vi "Create Actor Object.vi"(8 "error in (no error)":errorcluster, 10 "Object Name":string, 11 "CS++Factory in":refnum<class "CS++Factory.lvclass">) -> (0 "error out":errorcluster, 1 "Attributes found?":bool, 2 "C++BaseActor":refnum<class "CS++BaseActor.lvclass">, 3 "CS++Factory out":refnum<class "CS++Factory.lvclass">)   [LabVIEW 2013, in "CS++BaseClasses.lvlib" / "CS++Factory.lvclass"]
doc: "Create an actor object by name. Object name is a kind of reference to attribute initialization data."
uses:
  CS++Factory.lvclass
  Actors/CS++BaseActor/CS++BaseActor.lvclass
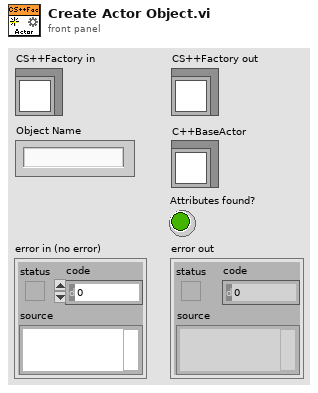
[diagram p1: front panel]
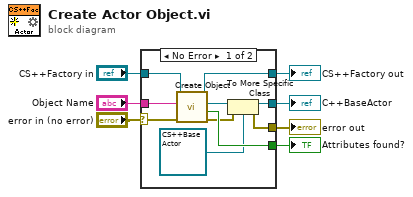
[diagram p0: block diagram]
diagram:
  n1 = case shown="No Error" "error in (no error)" {
    selector: "error in (no error)" -> [w11 w18]
    tunnel: "CS++Factory in" -> [w17 w19]
    tunnel: "Object Name" -> [w16 _]
    tunnel: [w15 w19] -> w5
    tunnel: [w14 _] -> w4
    tunnel: [w9 _] -> w3
    tunnel: [w8 w18] -> w2
    frame No Error {
      n2 = call "Create Object.vi"("error in (no error)"=w11, "Object Name"=w16, "CS++Factory in"=w17) -> ("error out"=w13:errorcluster, "Attributes found?"=w14:bool, "LabVIEW Object"=w12:refnum<class>, "CS++Factory out"=w15:refnum<class "CS++Factory.lvclass">)  [unwired: 5 in]
      n3 = To More Specific Class(target class=refnum<class "CS++BaseActor.lvclass"> refnum ("CS++BaseActor.lvlib:CS++BaseActor.lvclass"), reference=w12, error in=w13) -> (specific class reference=w9:refnum<class "CS++BaseActor.lvclass">, error out=w8:errorcluster)
    }
    frame Error {
    }
  }
  "error out" <- w2
  "CS++Factory out" <- w5
  "C++BaseActor" <- w3
  "Attributes found?" <- w4
